vi "膨脹閥.vi"() -> ()   [LabVIEW 2022 SP3]
uses:
  <vilib>/httpClient/LabVIEWHTTPClient.lvlib
panel:
  out "偏移量":dbl
  out "開度最小值":dbl
  out "HI":dbl
  out "LO":dbl
  out "壓力設定":dbl
  out "PT-1":dbl
  out "自動手動":bool
  in  "激磁":bool
  in  "位置滑條":dbl(slide) min=0.0 max=400.0 step=1.0 scale=0.0..400.0
  out "目前位置":dbl
  in  "START":bool
  out "開度輸入":dbl
  out "關按鈕":bool caption="Boolean"
  out "開按鈕":bool caption="Boolean"
  in  "開關切換":bool
  # "勘等恢"
  # "開"
  # "關"
  # "開度輸入"
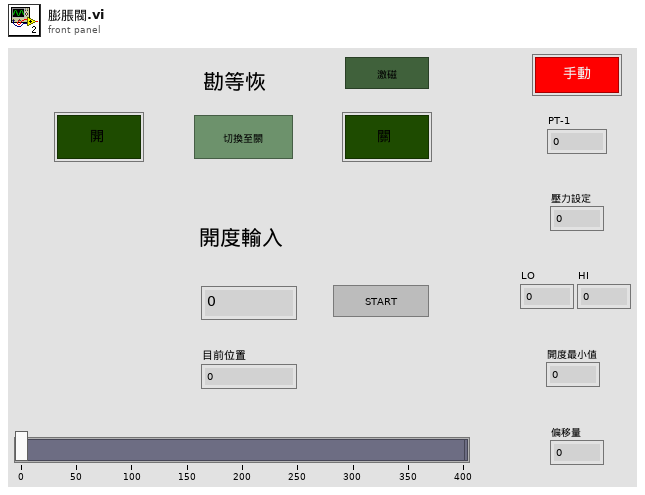
[diagram p1: front panel]
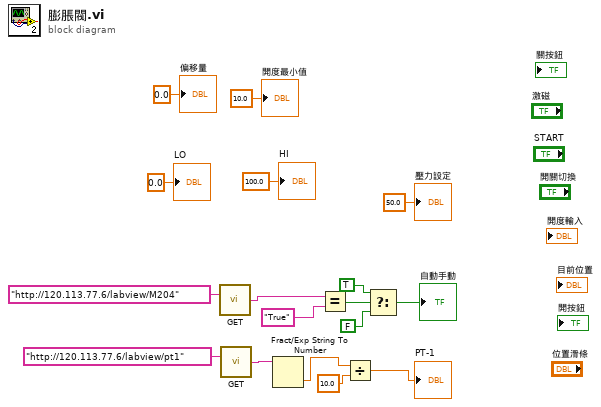
[diagram p0: block diagram]
diagram:
  n1 = call <vilib>:"GET.vi"("url"="http://120.113.77.6/labview/M204") -> ("body"=w7:string)  [unwired: 11 in, 3 out]
  n2 = call <vilib>:"GET.vi"("url"="http://120.113.77.6/labview/pt1") -> ("body"=w15:string)  [unwired: 11 in, 3 out]
  n3 = Fract/Exp String To Number(string=w15) -> (number=w13:dbl)  [unwired: 3 in, 1 out]
  n4 = Equal?(x=w7, y="True") -> (x = y?=w6:bool)
  "自動手動" <- w6
  n5 = Divide(x=w13, y=10.0) -> (x/y=→"PT-1":dbl)
  n6 = Select(t=TRUE, s=w6, f=FALSE) -> ()  [unwired: 1 out]
  "壓力設定" <- 50.0 ("壓力設定")
  "LO" <- 0.0 ("LO")
  "HI" <- 100.0 ("HI")
  "開度最小值" <- 10.0 ("開度最小值")
  "偏移量" <- 0.0 ("偏移量")
